vi "Assert Equal.vi"(5 "Expected":variant, 7 "Message (\"\")":string, 8 "error in (no error)":errorcluster, 10 "Actual":variant) -> (0 "error out":errorcluster)   [LabVIEW 2017, in "Transparent Assertions.lvlib" / "Assertions.lvlib"]
doc: "Asserts that two values are equal. Returns an error if the assertion fails, and optionally appends a custom message to the error."
uses:
  Assertions.lvlib
  Constraints/IsEqual/IsEqual.lvclass
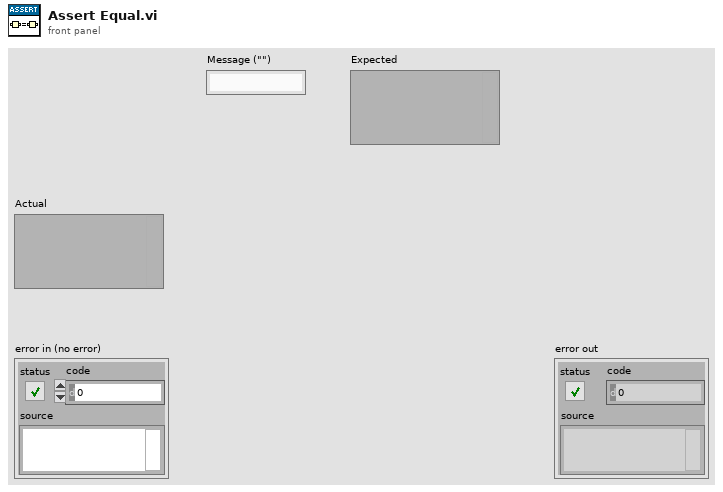
[diagram p1: front panel]
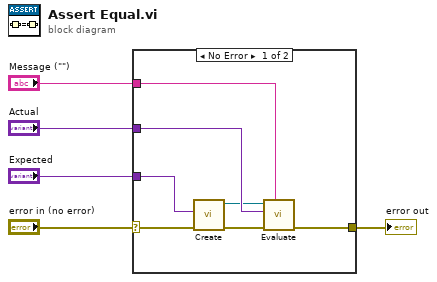
[diagram p0: block diagram]
diagram:
  n1 = case shown="No Error" "error in (no error)" {
    selector: "error in (no error)" -> [w9 w13]
    tunnel: "Actual" -> [w12 _]
    tunnel: [w11 w13] -> w5
    tunnel: "Message (\"\")" -> [w10 _]
    tunnel: "Expected" -> [w6 _]
    frame No Error {
      n2 = call "Create.vi"("error in (no error)"=w9, "Expected"=w6) -> ("error out"=w8:errorcluster, "IsEqual"=w7:refnum<class "IsEqual.lvclass">)  [unwired: 8 in]
      n3 = call-dynamic "Evaluate.vi"("Message (\"\")"=w10, "error in (no error)"=w8, "Actual"=w12, "Constraint in"=w7) -> ("error out"=w11:errorcluster)  [unwired: 6 in, 1 out]
    }
    frame Error {
    }
  }
  "error out" <- w5
